vi "cluster.vi"() -> ()   [LabVIEW 2015]
panel:
  in  "Cluster":cluster{bool, bool, bool, bool}
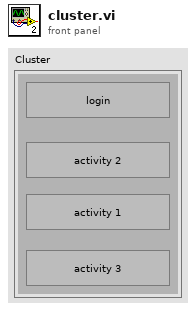
[diagram p1: front panel]
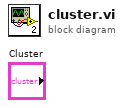
[diagram p0: block diagram]
diagram:
